vi "Controllers_PIDFemto.vi"(6 "Offset (0) / 1E-5 V":dbl, 8 "Error in":errorcluster, 11 "Task In":refnum<k21>) -> (0 "Error Out":errorcluster, 2 "RT Femto / V":dbl, 3 "Task Out":refnum<k21>)   [LabVIEW 2023]
uses:
  <vilib>/DAQmx/read.llb/DAQmx Read (Analog 1D DBL NChan 1Samp).vi
  <vilib>/DAQmx/miscellaneous.llb/DAQmx Fill In Error Info.vi
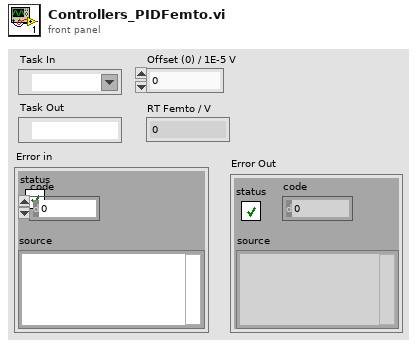
[diagram p1: front panel]
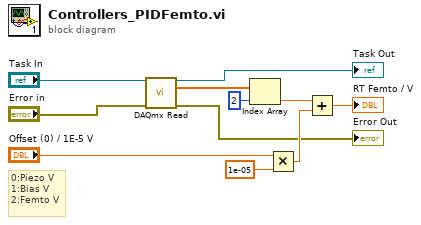
[diagram p0: block diagram]
diagram:
  # "0:Piezo V\n1:Bias V\n2:Femto V"
  n1 = call-poly <vilib>:"DAQmx Read.vi"("task/channels in"="Task In", "error in"="Error in") -> ("task out"=→"Task Out":refnum<k21>, "data"=w7:dbl[], "error out"=→"Error Out":errorcluster)  [unwired: 11 in]
  n2 = Index Array(array=w7, index=2) -> (element=w6:dbl)
  n3 = Multiply(x="Offset (0) / 1E-5 V", y=1e-05) -> (x*y=w4:dbl)
  n4 = Add(x=w6, y=w4) -> (x+y=→"RT Femto / V":dbl)
